vi "SetComparisonType.vi"(8 "error in":errorcluster, 10 "ComparisonType":T1, 11 "RangeMeasureLimit in":refnum<class "RangeMeasureLimit.lvclass">) -> (0 "error out":errorcluster, 3 "RangeMeasureLimit out":refnum<class "RangeMeasureLimit.lvclass">)   [LabVIEW 2021, in "ProligentXMLGenerator.lvlib" / "RangeMeasureLimit.lvclass"]
doc: "Real Measure Limit Comparison Type"
uses:
  RangeMeasureLimit.lvclass
  RangeMeasureLimit.lvclass/RangeMeasureLimit.ctl
  ComparisonType.ctl
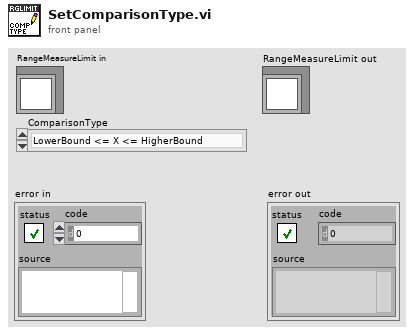
[diagram p1: front panel]
types:
  T1 = typedef "ProligentXMLGenerator.lvlib/RangeMeasureLimit.lvclass/ComparisonType.ctl" = enum16{"LowerBound <= X <= HigherBound", "LowerBound < X <= HigherBound", "LowerBound <= X < HigherBound", "LowerBound < X < HigherBound", "LowerBound <= X", "LowerBound < X", "X <= HigherBound", "X < HigherBound", "X == HigherBound", "X != HigherBound", "X <= LowerBound OR HigherBound <= X", "X < LowerBound OR HigherBound <= X", "X <= LowerBound OR HigherBound < X", "X < LowerBound OR HigherBound < X"}
  T2 = typedef "ProligentResultProcessor.lvlib/RangeMeasureLimit.lvclass/Data.ctl" = cluster{"ComparisonType":T3}
  T3 = typedef "ProligentResultProcessor.lvlib/RangeMeasureLimit.lvclass/ComparisonType.ctl" = enum16{"LowerBound <= X <= HigherBound", "LowerBound < X <= HigherBound", "LowerBound <= X < HigherBound", "LowerBound < X < HigherBound", "LowerBound <= X", "LowerBound < X", "X <= HigherBound", "X < HigherBound", "X == HigherBound", "X != HigherBound", "X <= LowerBound OR HigherBound <= X", "X < LowerBound OR HigherBound <= X", "X <= LowerBound OR HigherBound < X", "X < LowerBound OR HigherBound < X"}
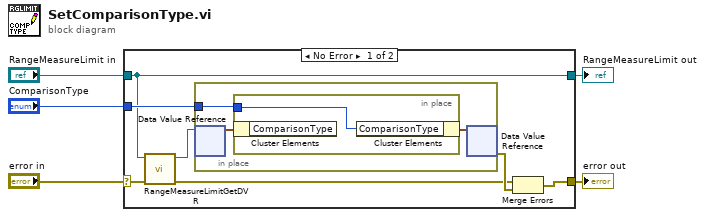
[diagram p0: block diagram]
diagram:
  n1 = case shown="No Error" "error in" {
    selector: "error in" -> [w8 w17]
    tunnel: "RangeMeasureLimit in" -> [w7 w18]
    tunnel: [w11 w17] -> w1
    tunnel: "ComparisonType" -> [w10 _]
    tunnel: [w7 w18] -> w2
    frame No Error {
      n2 = call "RangeMeasureLimitGetDVR.vi"("error in"=w8, "RangeMeasureLimit"=w7) -> ("error out"=w6:errorcluster, "DVRReference"=w12:refnum<data-value>)  [unwired: 8 in]
      n3 = in-place "In Place Element Structure" {
        in-place-border: w10 -> [w15]
        n4 = in-place-dvr #1(w12) -> (w14:T2)  [unwired: 1 out]
        n5 = in-place "In Place Element Structure" {
          in-place-border: w15 -> [w16]
          n6 = in-place-cluster #2(w14) -> ()  [unwired: 1 out]
          n7 = in-place-cluster #2("ComparisonType"=w16) -> (w13:T2)
        }
        n8 = in-place-dvr #1(w13) -> (w9:errorcluster)  [unwired: 1 out]
      }
      n9 = Merge Errors(w6, w9) -> (w11:errorcluster)
    }
    frame Error {
    }
  }
  "error out" <- w1
  "RangeMeasureLimit out" <- w2
